vi "Post-Request.vi"(8 "error in (no error)":errorcluster, 10 "http-method in":refnum<class "http-client.lvclass">, 11 "REST Client in":refnum<class "REST Client.lvclass">) -> (0 "error out":errorcluster, 3 "REST Client out":refnum<class "REST Client.lvclass">)   [LabVIEW 2020, in "REST Client.lvlib" / "REST Client.lvclass"]
uses:
  REST Client.lvclass
  http-client/http-client.lvclass
  REST Client.lvclass/REST Client.ctl
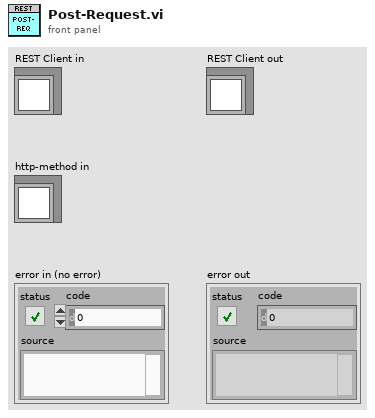
[diagram p1: front panel]
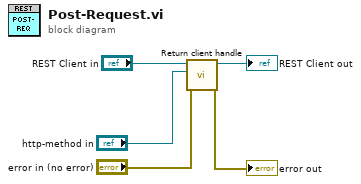
[diagram p0: block diagram]
diagram:
  n1 = call "Return client handle.vi"("error in (no error)"="error in (no error)", "http-client"="http-method in", "REST Client in"="REST Client in") -> ("error out"=→"error out":errorcluster, "REST Client out"=→"REST Client out":refnum<class "REST Client.lvclass">)  [unwired: 7 in]
